vi "Camera Info Grab.vi"() -> (2 "Physical Paths":string[](array[string]), 3 "Logical Paths":string[](array[string]))   [LabVIEW 2015]
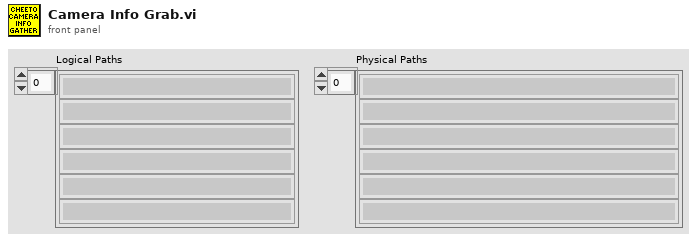
[diagram p1: front panel]
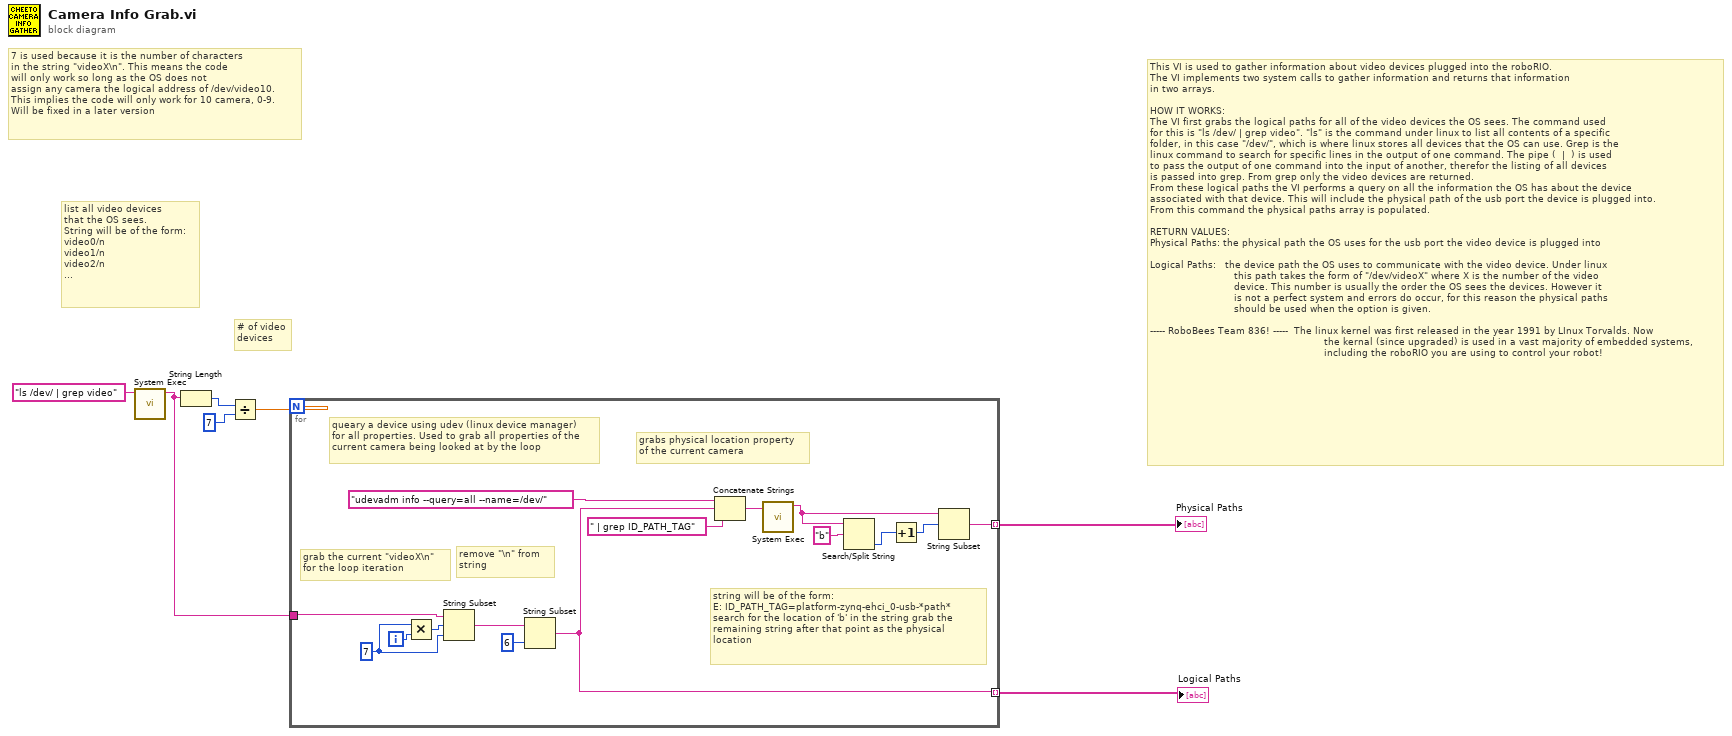
[diagram p0: block diagram]
diagram:
  # "This VI is used to gather information about video devices plugged into the roboRIO.\nThe VI implements two system calls to gather information and returns that information\nin two arrays.\n\nHOW IT WORKS:\nThe VI first grabs the logical paths for all of the video devices the OS sees. The command used\nfor this is \"ls /dev/ | grep video\". \"ls\" is the command under linux to list all contents of a specific\nfolder, in this case \"/dev/\", which is where linux stores all devices that the OS can use. Grep is the\nlinux command to search for specific lines in the output of one command. The pipe (  |  ) is used \nto pass the output of one command into the input of another, therefor the listing of all devices\nis passed into grep. From grep only the video devices are returned.\nFrom these logical paths the VI performs a query on all the information the OS has about the device\nassociated with that device. This will include the physical path of the usb port the device is plugged into.\nFrom this command the physical paths array is populated. \n\nRETURN VALUES:\nPhysical Paths: the physical path the OS uses for the usb port the video device is plugged into\n\nLogical Paths:   the device path the OS uses to communicate with the video device. Under linux\n                            this path takes the form of \"/dev/videoX\" where X is the number of the video\n                            device. This number is usually the order the OS sees the devices. However it\n                            is not a perfect system and errors do occur, for this reason the physical paths\n                            should be used when the option is given.\n\n----- RoboBees Team 836! -----  The linux kernel was first released in the year 1991 by LInux Torvalds. Now\n                                                          the kernal (since upgraded) is used in a vast majority of embedded systems,\n                                                          including the roboRIO you are using to control your robot!"
  # "7 is used because it is the number of characters\nin the string \"videoX\\n\". This means the code\nwill only work so long as the OS does not\nassign any camera the logical address of /dev/video10.\nThis implies the code will only work for 10 camera, 0-9.\nWill be fixed in a later version"
  # "list all video devices\nthat the OS sees.\nString will be of the form:\nvideo0/n\nvideo1/n\nvideo2/n\n..."
  # "# of video\ndevices"
  n1 = call <vilib>:"System Exec.vi"("command line"="ls /dev/ | grep video") -> ("standard output"=w4:string)  [unwired: 7 in, 3 out]
  n2 = String Length(string=w4) -> (length=w6:i32)
  n3 = Divide(x=w6, y=7) -> (x/y=w1:dbl)
  n4 = for {
    N: w1 -> [_]
    tunnel: w4 -> [w19]
    tunnel: [w8] -> w3 mode=indexing
    tunnel: [w9] -> w2 mode=indexing
    i -> [w18]
    w22 = 7 ("length (rest)")
    # "string will be of the form:\nE: ID_PATH_TAG=platform-zynq-ehci_0-usb-*path*\nsearch for the location of 'b' in the string grab the \nremaining string after that point as the physical\nlocation"
    # "grabs physical location property\nof the current camera"
    # "queary a device using udev (linux device manager)\nfor all properties. Used to grab all properties of the\ncurrent camera being looked at by the loop"
    # "remove \"\\n\" from\nstring"
    # "grab the current \"videoX\\n\"\nfor the loop iteration"
    n5 = Multiply(x=w22, y=w18) -> (x*y=w21:i32)
    n6 = String Subset(string=w19, offset (0)=w21, length (rest)=w22) -> (substring=w17:string)
    n7 = String Subset(string=w17, length (rest)=6 ("length (rest)")) -> (substring=w8:string)  [unwired: 1 in]
    n8 = Concatenate Strings("udevadm info --query=all --name=/dev/" ("command line"), w8, " | grep ID_PATH_TAG" ("string")) -> (w14:string)
    n9 = call <vilib>:"System Exec.vi"("command line"=w14) -> ("standard output"=w10:string)  [unwired: 7 in, 3 out]
    n10 = Search/Split String(string=w10, search string/char (-)="b") -> (offset of match=w12:i32)  [unwired: 1 in, 2 out]
    n11 = Increment(x=w12) -> (x+1=w11:i32)
    n12 = String Subset(string=w10, offset (0)=w11) -> (substring=w9:string)  [unwired: 1 in]
  }
  "Logical Paths" <- w3
  "Physical Paths" <- w2
